vi "Color Sensor V3 Config ProxSensor LED.vi"(0 "ColorSensorDevRef":T3={"I2CDevRef"={"DevStatus"={"status"=FALSE, "code"=0, "source"=""}, "Device Address"=0, "Handle"=0, "I2C Bus"=enum."Invalid"}} {"I2CDevRef"."Device Address" format="%.0x"}, 5 "LEDPulseFreq":T2, 7 "LEDCurrent":T1, 9 "Pulses":u8, 11 "error in (no error)":errorcluster) -> (4 "ColorSensorDevRef out":T3={"I2CDevRef"={"DevStatus"={"status"=FALSE, "code"=0, "source"=""}, "Device Address"=0, "Handle"=0, "I2C Bus"=enum."Invalid"}} {"I2CDevRef"."Device Address" format="%.0x"}, 15 "error out":errorcluster)   [LabVIEW 2023]
uses:
  Typedef/Color Sensor V3 DevRef.ctl
  <vilib>/Rock Robotics/WPI/I2C/WPI_I2CDevRef.ctl
  <vilib>/Rock Robotics/SystemInterfaces/i2clib/i2c_bus.ctl
  Typedef/Color Sensor V3 LEDPulseFreq.ctl
  Typedef/Color Sensor V3 LEDCurrent.ctl
  Typedef/Color Sensor V3 Registers.ctl
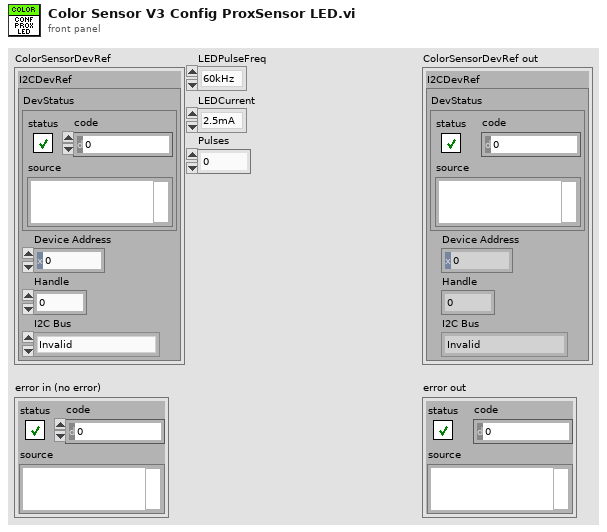
[diagram p1: front panel]
types:
  T1 = typedef "Color Sensor V3 LEDCurrent.ctl" = enum8{"2.5mA", "5.0mA", "10mA", "25mA", "50mA", "75mA", "100mA", "125mA"}
  T2 = typedef "Color Sensor V3 LEDPulseFreq.ctl" = enum16{"60kHz", "70kHz", "80kHz", "90kHz", "100kHz"}
  T3 = typedef "Color Sensor V3 DevRef.ctl" = cluster{"I2CDevRef":T4}
  T4 = typedef "WPI_I2CDevRef.ctl" = cluster{"DevStatus":errorcluster, "Device Address":u8, "Handle":i32, "I2C Bus":T5}
  T5 = typedef "i2c_bus.ctl" = enum16{"I2C On-Board", "I2C MXP", "Invalid"}
  T6 = typedef "Color Sensor V3 Registers.ctl" = enum16{"MainCtrl", "ProximitSensorLED", "ProximitySensorPulse", "ProximitySensorRate", "LightSensorMeasurementRate", "LightSensorGainRegister", "PartIDRegister", "MainStatus", "ProximityData", "ProximityData1", "InfraredData", "InfraredData1", "InfraredData2", "GreenData", "GreenData1", "GreenData2", "BlueData", "BlueData1", "BlueData2", "RedData", "RedData1", "RedData2"}
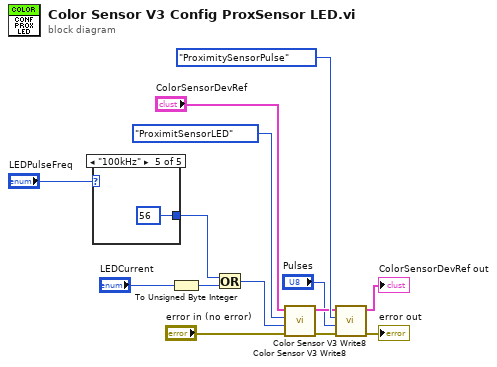
[diagram p0: block diagram]
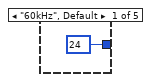
[diagram p2: hidden frame]
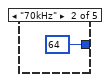
[diagram p3: hidden frame]
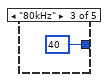
[diagram p4: hidden frame]
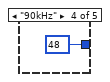
[diagram p5: hidden frame]
diagram:
  n1 = case shown="\"100kHz\"" "LEDPulseFreq" {
    tunnel: [u8 24 ("Data") u8 64 ("Data") u8 40 ("Data") u8 48 ("Data") u8 56 ("Data")] -> w10
    frame "60kHz", Default {
    }
    frame "70kHz" {
    }
    frame "80kHz" {
    }
    frame "90kHz" {
    }
    frame "100kHz" {
    }
  }
  n2 = To Unsigned Byte Integer(number="LEDCurrent") -> (unsigned 8bit integer=w8:u8)
  n3 = Or(x=w10, y=w8) -> (x .or. y?=w7:u8)
  n4 = call "Color Sensor V3 Write8.vi"("error in (no error)"="error in (no error)", "Data"=w7, "Registers"=Color_Sensor_V3_Registers."ProximitSensorLED", "ColorSensorDevRef"="ColorSensorDevRef") -> ("error out"=w4:errorcluster, "ColorSensorDevRef out"=w5:T3)  [unwired: 6 in]
  n5 = call "Color Sensor V3 Write8.vi"("error in (no error)"=w4, "Data"="Pulses", "Registers"=Color_Sensor_V3_Registers."ProximitySensorPulse", "ColorSensorDevRef"=w5) -> ("error out"=→"error out":errorcluster, "ColorSensorDevRef out"=→"ColorSensorDevRef out":T3)  [unwired: 6 in]
